vi "Matches.vi"(8 "error in (no error)":errorcluster, 10 "Actual":variant, 11 "Is Greater Than in":refnum<class "Is Greater Than.lvclass">) -> (0 "error out":errorcluster, 2 "Result":bool, 3 "Is Greater Than out":refnum<class "Is Greater Than.lvclass">)   [LabVIEW 2017, in "Transparent Assertions.lvlib" / "Constraints.lvlib" / "Is Greater Than.lvclass"]
doc: "Evaluates the constraint for <B>Actual</B>. Returns true if the constraint is met."
uses:
  Is Greater Than.lvclass
  Is Greater Than.lvclass/Is Greater Than.ctl
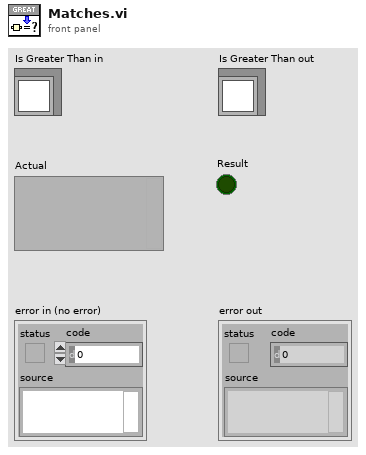
[diagram p1: front panel]
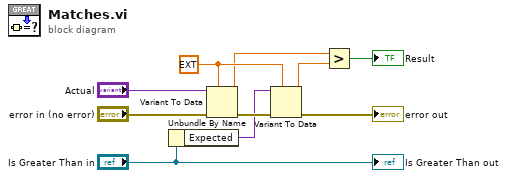
[diagram p0: block diagram]
diagram:
  w3 = ext 0.0
  n1 = Unbundle By Name("Is Greater Than in") -> ("Expected"=w4:variant)
  n2 = Variant To Data(error in="error in (no error)", type=w3, Variant="Actual") -> (data=w2:ext, error out=w6:errorcluster)
  n3 = Variant To Data(error in=w6, type=w3, Variant=w4) -> (data=w1:ext, error out=→"error out":errorcluster)
  n4 = Greater?(x=w2, y=w1) -> (0:→"Result":bool)
  "Is Greater Than out" <- "Is Greater Than in"
